vi "Read Stage Homed.vi"(8 "error in (no error)":errorcluster, 11 "Sync 2-Axis Stage Controller in":refnum<class "Sync 2-Axis Stage Controller.lvclass">) -> (0 "error out":errorcluster, 1 "Y-Axis Homed":bool, 2 "X-Axis Homed":bool, 3 "Sync 2-Axis Stage Controller out":refnum<class "Sync 2-Axis Stage Controller.lvclass">)   [LabVIEW 2022 SP3, in "Sync 2-Axis Stage Controller.lvclass"]
uses:
  Sync 2-Axis Stage Controller.lvclass
  Sync 2-Axis Stage Controller.lvclass/Sync 2-Axis Stage Controller.ctl
  Axis Objects/iMotion Controller/iMotion Controller.lvclass
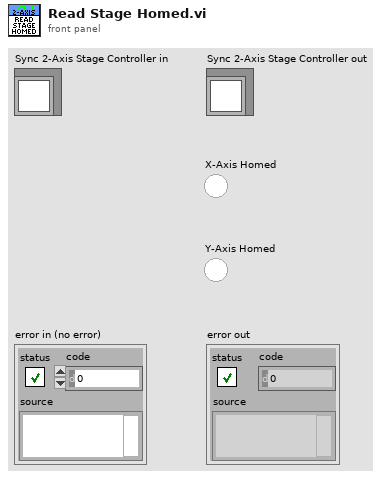
[diagram p1: front panel]
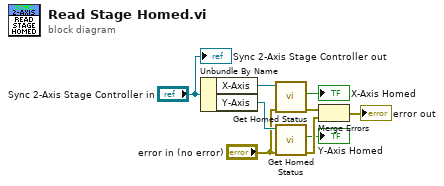
[diagram p0: block diagram]
diagram:
  n1 = Unbundle By Name("Sync 2-Axis Stage Controller in") -> ("X-Axis"=w9:refnum<class "iMotion Controller.lvclass">, "Y-Axis"=w8:refnum<class "iMotion Controller.lvclass">)
  n2 = call-dynamic "Get Homed Status.vi"("error in (no error)"="error in (no error)", "iMotion Controller in"=w9) -> ("error out"=w4:errorcluster, "Homed"=→"X-Axis Homed":bool)  [unwired: 7 in, 1 out]
  n3 = call-dynamic "Get Homed Status.vi"("error in (no error)"="error in (no error)", "iMotion Controller in"=w8) -> ("error out"=w7:errorcluster, "Homed"=→"Y-Axis Homed":bool)  [unwired: 7 in, 1 out]
  n4 = Merge Errors(w4, w7) -> (→"error out":errorcluster)
  "Sync 2-Axis Stage Controller out" <- "Sync 2-Axis Stage Controller in"
